vi "Magazine_Execute.vi"   [LabVIEW 2020]
uses:
  Utility VIs/Basic_Motor_Modes.ctl
  Globals/Magazine_Globals.vi
  Globals/Sensor_Values.vi
types:
  T1 = typedef "Basic_Motor_Modes.ctl" = enum16{"Percent_Voltage", "Speed_Control", "Position_Control", "Current"}
  T2 = typedef "Magazine_Cluster.ctl" = cluster{"Control_States":T3, "Manual_Magazine":dbl, "Load_Magazine":bool, "Firing_Magazine":bool, "Load/Firing Velocity":dbl}
  T3 = typedef "Magazine_Control_States.ctl" = enum16{"No-Op", "Manual_%Vbus", "Manual_Speed_Control", "Load", "Firing"}
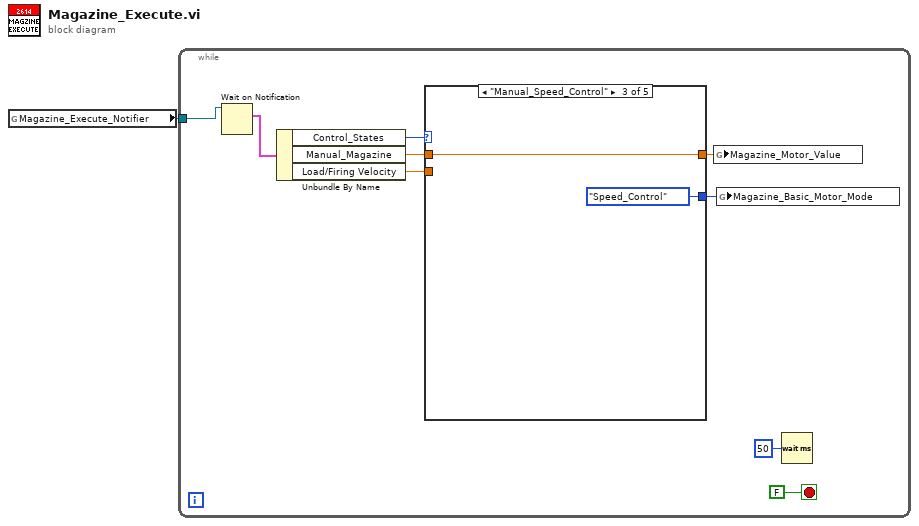
[diagram p0: block diagram]
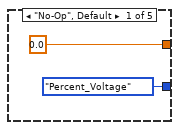
[diagram p2: hidden frame]
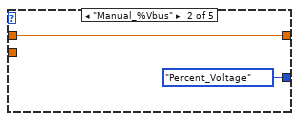
[diagram p3: hidden frame]
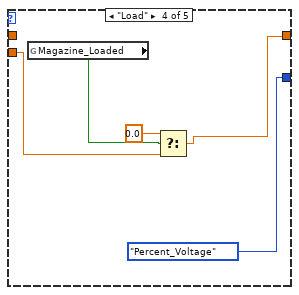
[diagram p4: hidden frame]
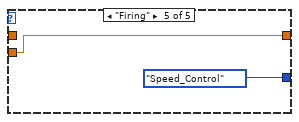
[diagram p5: hidden frame]
diagram:
  n1 = global read "Magazine_Globals.vi" "Magazine_Execute_Notifier"() -> (w1:refnum<notifier>)
  n2 = while {
    tunnel: w1 -> [w10]
    stop <- FALSE stop-if-true
    n3 = Wait on Notification(notifier=w10) -> (notification=w7:T2)  [unwired: 3 in, 3 out]
    n4 = Unbundle By Name(w7) -> ("Control_States"=w6:T3, "Manual_Magazine"=w5:dbl, "Load/Firing Velocity"=w2:dbl)
    n5 = case shown="\"Manual_Speed_Control\"" w6 {
      tunnel: [0.0 w14 w15 w17 w22] -> w4
      tunnel: w5 -> [_ w14 w15 _ _]
      tunnel: [Basic_Motor_Modes."Percent_Voltage" ("Basic_Motor_Mode") Basic_Motor_Modes."Percent_Voltage" ("Basic_Motor_Mode") Basic_Motor_Modes."Speed_Control" ("Basic_Motor_Mode") Basic_Motor_Modes."Percent_Voltage" ("Basic_Motor_Mode") Basic_Motor_Modes."Speed_Control" ("Basic_Motor_Mode")] -> w3
      tunnel: w2 -> [_ _ _ w19 w22]
      frame "No-Op", Default {
      }
      frame "Manual_%Vbus" {
      }
      frame "Manual_Speed_Control" {
      }
      frame "Load" {
        n6 = global read "Sensor_Values.vi" "Magazine_Loaded"() -> (w20:bool)
        n7 = Select(t=0.0, s=w20, f=w19) -> (s? t:f=w17:dbl)
      }
      frame "Firing" {
      }
    }
    n8 = global write "Magazine_Globals.vi" "Magazine_Motor_Value"(w4) -> ()
    n9 = global write "Magazine_Globals.vi" "Magazine_Basic_Motor_Mode"(w3) -> ()
    n10 = Wait (ms)(milliseconds to wait=u32 50) -> ()  [unwired: 1 out]
  }
